vi "数据表比对.vi"(6 "table输入 3":string(combo), 8 "error in (no error)":errorcluster, 9 "table输入 2":string(combo), 10 "仪器日志参数":string, 11 "table输入":string(combo)) -> (0 "error out":errorcluster, 2 "待发送第一条数据":string[](array[string]), 3 "待发送数据":string[][](table), 4 "获取有效数据":string[][](array[string]))   [LabVIEW 2016]
panel:
  out "获取有效数据 3":string[][](array[string])
  out "获取有效数据 2":string[][](array[string])
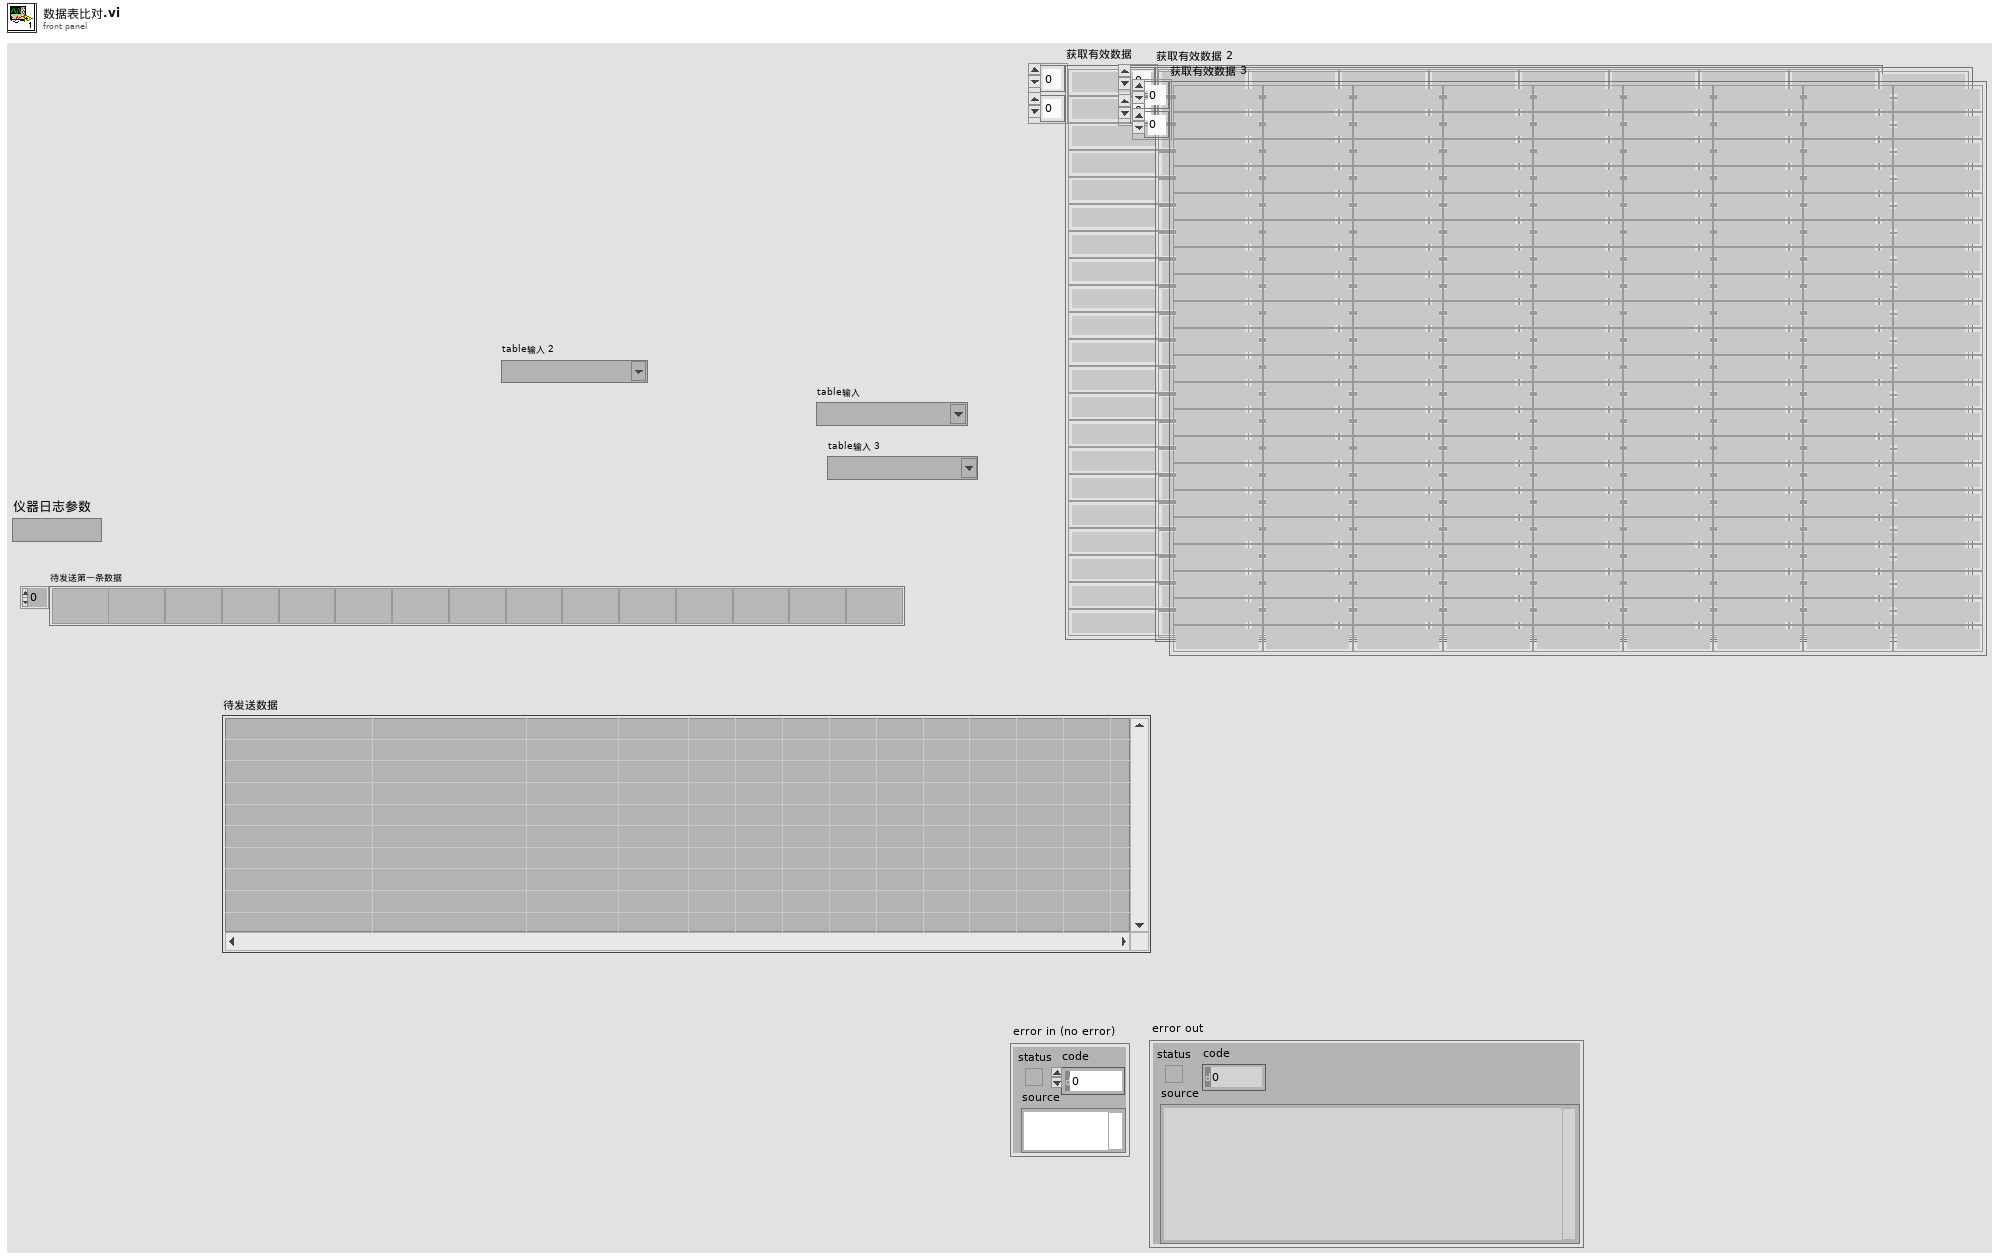
[diagram p1: front panel]
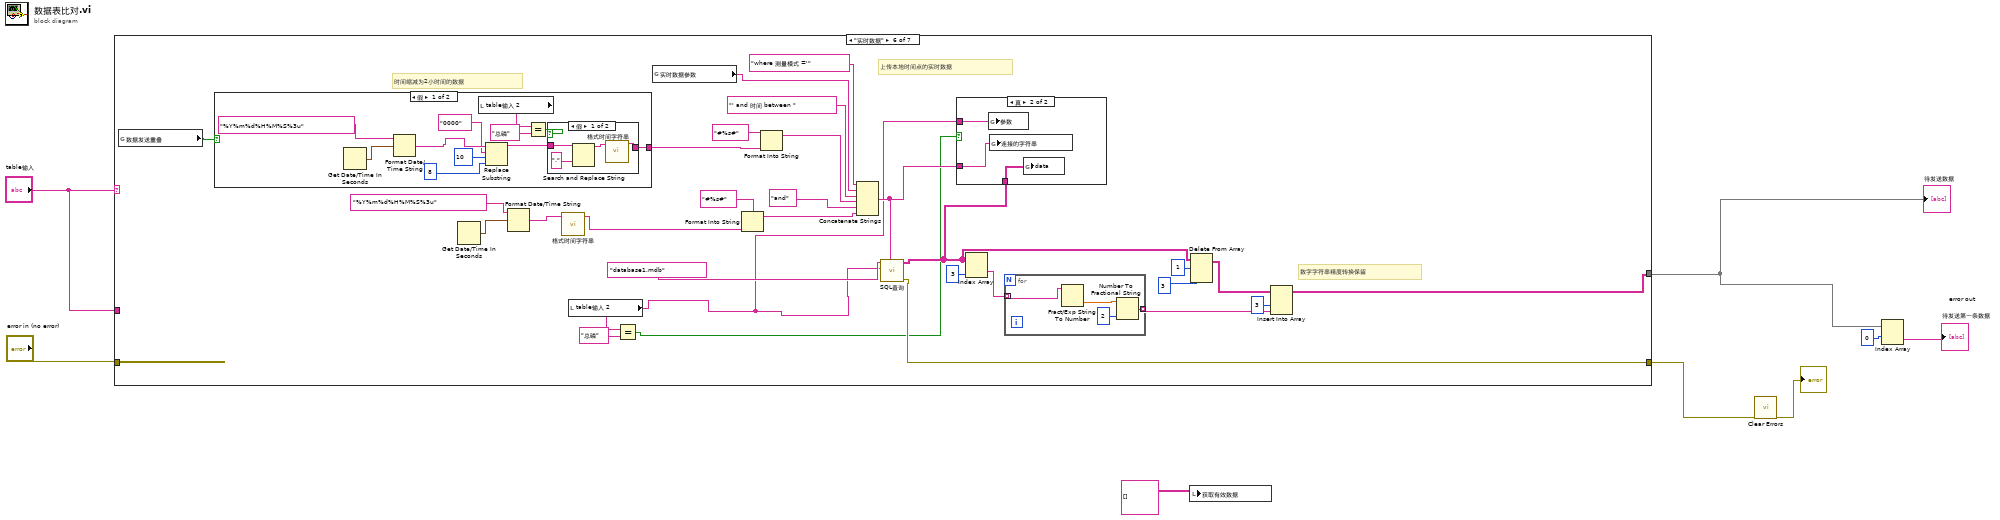
[diagram p0: block diagram]
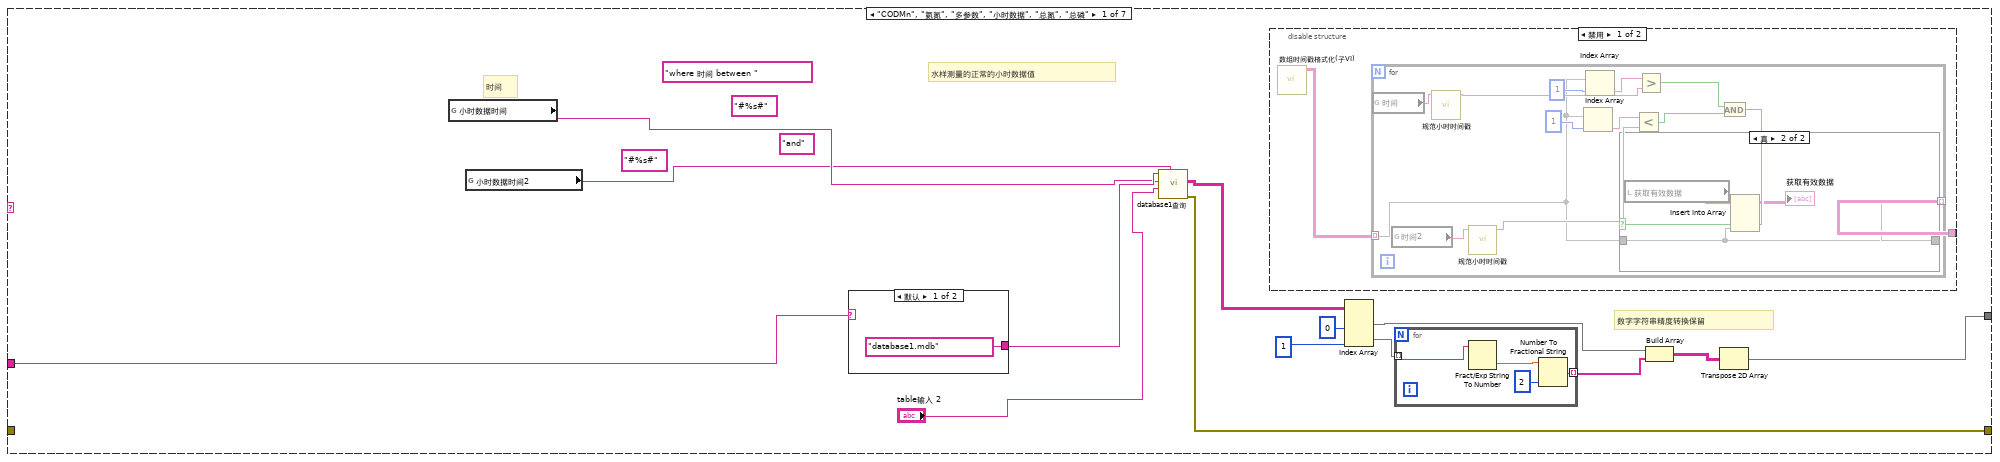
[diagram p2: hidden frame]
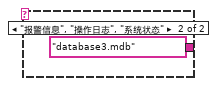
[diagram p5: hidden frame]
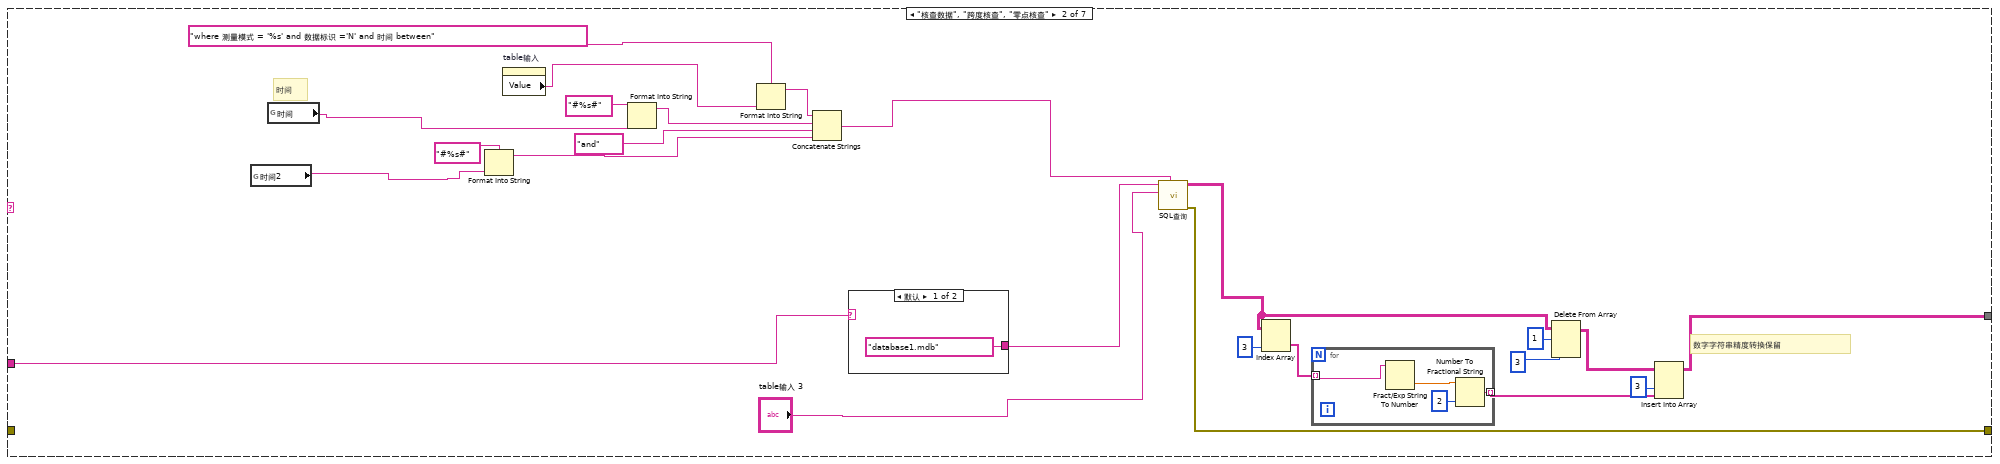
[diagram p6: hidden frame]
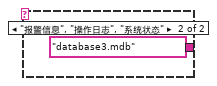
[diagram p7: hidden frame]
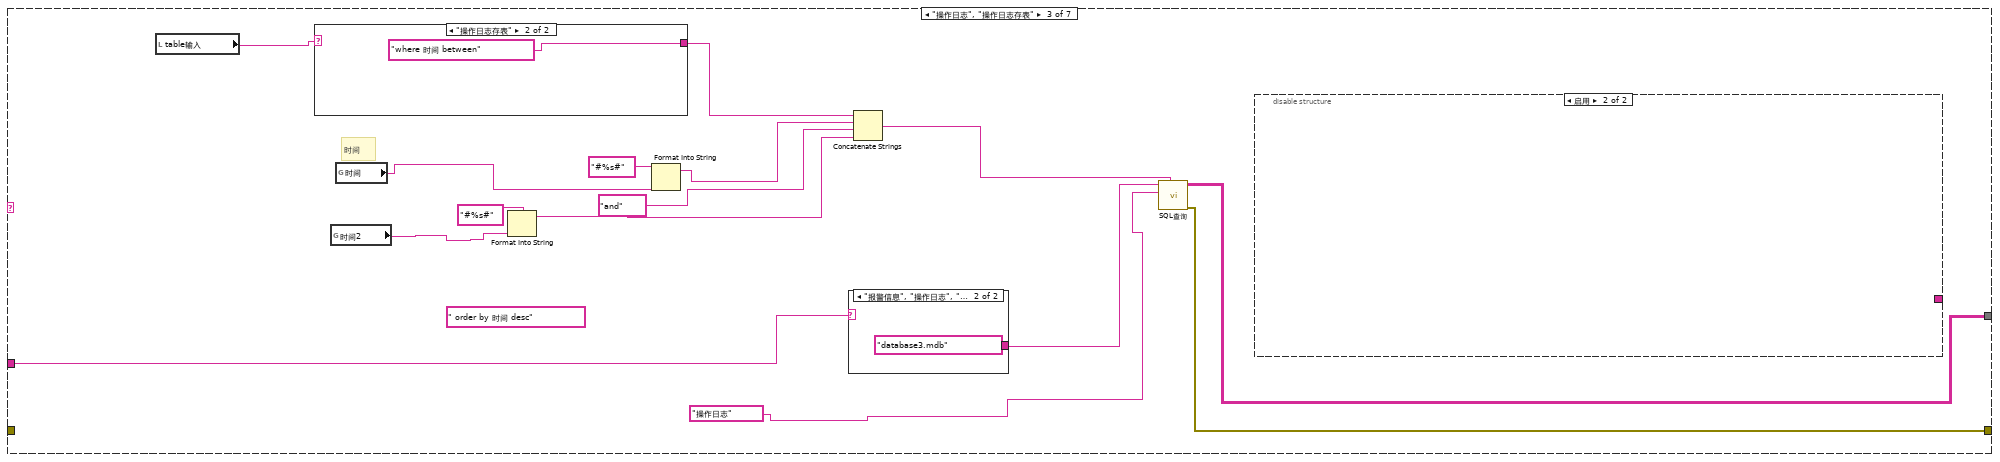
[diagram p8: hidden frame]
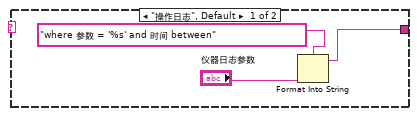
[diagram p9: hidden frame]
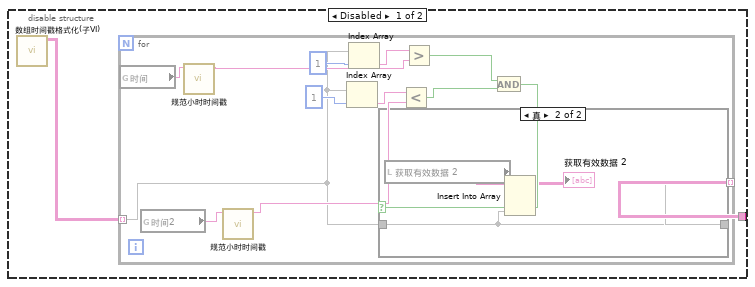
[diagram p10: hidden frame]
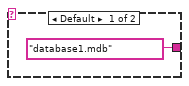
[diagram p12: hidden frame]
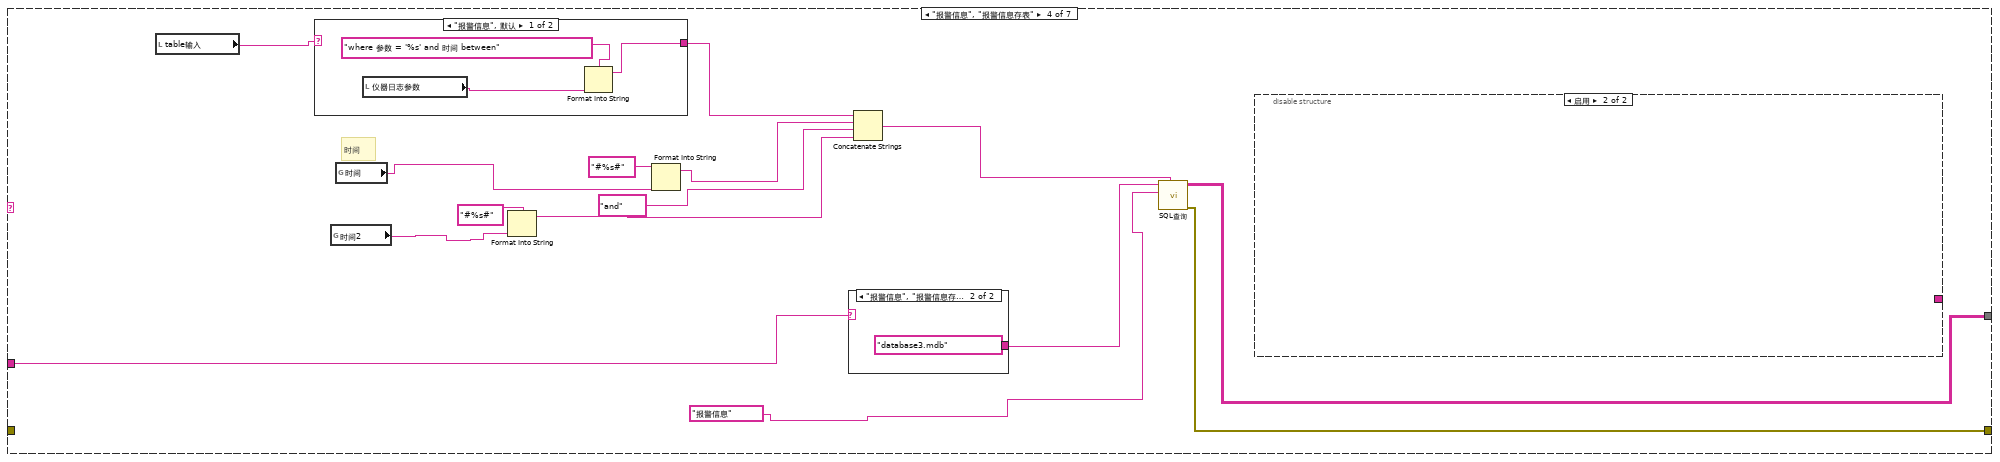
[diagram p13: hidden frame]
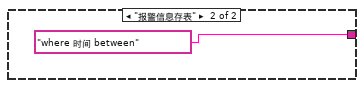
[diagram p14: hidden frame]
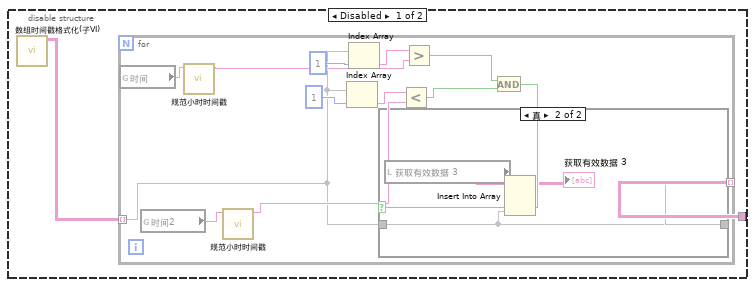
[diagram p15: hidden frame]
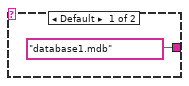
[diagram p17: hidden frame]
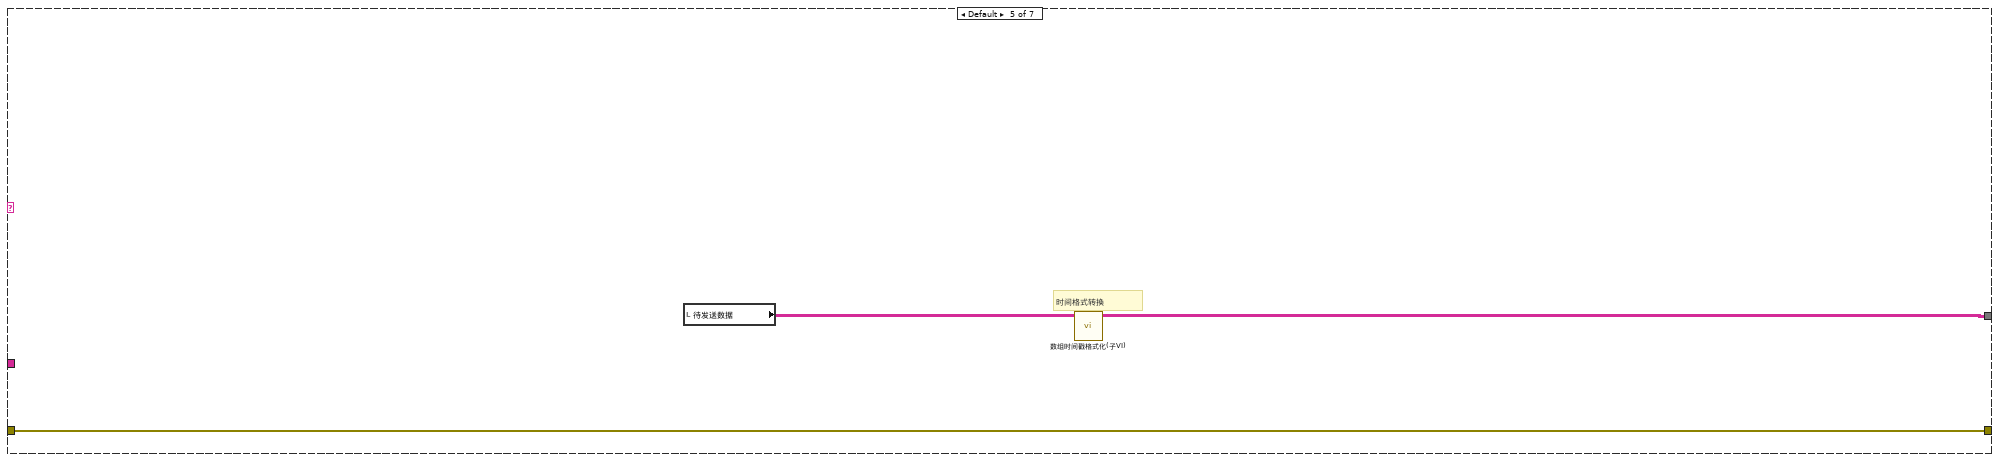
[diagram p18: hidden frame]
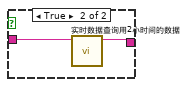
[diagram p20: hidden frame]
diagram:
  n1 = case shown="\"实时数据\"" "table输入" {
    tunnel: "error in (no error)" -> [_ _ _ _ w157 _ _]
    tunnel: [w19 w68 w89 w128 w157 w183 w221] -> w6
    tunnel: [w9 w47 w87 w126 w155 w165 w212] -> w2
    tunnel: "table输入" -> [w22 w70 w91 w130 _ _ _]
    frame "CODMn", "氨氮", "多参数", "小时数据", "总氮", "总磷" {
      (unwired) "and" ("字符串")
      (unwired) "#%s#" ("初始字符串")
      (unwired) "#%s#" ("初始字符串")
      (unwired) "where 时间 between " ("condition")
      # "数字字符串精度转换保留"
      # "水样测量的正常的小时数据值"
      # "时间"
      n2 = global read "全局 时间.vi" "小时数据时间"() -> (w18:string)
      n3 = global read "全局 时间2.vi" "小时数据时间2"() -> (w17:string)
      n4 = case shown="默认" w22 {
        tunnel: ["database1.mdb" ("database") "database3.mdb" ("database")] -> w21
        frame Default {
        }
        frame "报警信息", "操作日志", "系统状态" {
        }
      }
      n5 = call "database1查询.vi"("时间2"=w17, "table"="table输入 2", "时间1"=w18, "database"=w21) -> ("error out"=w19:errorcluster, "data"=w16:string[][])  [unwired: 4 in, 1 out]
      n6 = disable-structure shown="禁用" {
        disable-tunnel: [w27 _] -> _
        frame Disabled {
          n7 = call "数组时间戳格式化(子VI).vi"() -> ("待发送数据输出"=w28:string[][])  [unwired: 11 in]
          n8 = for {
            tunnel: w28 -> [w29] mode=indexing
            tunnel: [w31] -> w27 mode=indexing
            n9 = global read "全局 时间.vi" "时间"() -> (w35:string)
            n10 = global read "全局 时间2.vi" "时间2"() -> (w33:string)
            n11 = call "规范小时时间戳.vi"("字符串"=w35) -> ("result string"=w34:string)  [unwired: 10 in]
            n12 = call "规范小时时间戳.vi"("字符串"=w33) -> ("result string"=w32:string)  [unwired: 10 in]
            n13 = Index Array(array=w29, index=1 ("索引")) -> (element=w38:string)
            n14 = Index Array(array=w29, index=1 ("索引")) -> (element=w40:string)
            n15 = Less?(x=w38, y=w32) -> (x < y?=w37:bool)
            n16 = Greater?(x=w40, y=w34) -> (0:w36:bool)
            n17 = And(x=w36, y=w37) -> (x .and. y?=w30:bool)
            n18 = case shown="真" w30 {
              tunnel: w29 -> [_ w44]
              tunnel: [_ w44] -> w31
              frame False {
              }
              frame True {
                n19 = local read "获取有效数据"() -> (w43:string[][])
                n20 = Insert Into Array(array=w43, new element=w44) -> (→"获取有效数据":string[][])  [unwired: 2 in]
              }
            }
          }
        }
        frame Enabled {
        }
      }
      n21 = Index Array(array=w16, index (col) #1=0 ("禁用的索引 (列)"), index (col) #2=1 ("索引 (列)")) -> (element #1=w12:string[], element #2=w13:string[])  [unwired: 2 in]
      n22 = for {
        tunnel: w13 -> [w24] mode=indexing
        tunnel: [w23] -> w11 mode=indexing
        n23 = Fract/Exp String To Number(string=w24) -> (number=w25:dbl)  [unwired: 3 in, 1 out]
        n24 = Number To Fractional String(number=w25, precision (6)=i16 2 ("精度(6)")) -> (F-format string=w23:string)  [unwired: 2 in]
      }
      n25 = Build Array(w12, w11) -> (w10:string[][])
      n26 = Transpose 2D Array(2D array=w10) -> (transposed array=w9:string[][])
    }
    frame "核查数据", "跨度核查", "零点核查" {
      # "数字字符串精度转换保留"
      # "时间"
      n27 = global read "全局 时间2.vi" "时间2"() -> (w56:string)
      n28 = global read "全局 时间.vi" "时间"() -> (w57:string)
      n29 = Format Into String(format string="#%s#" ("初始字符串"), w56) -> (resulting string=w63:string)  [unwired: 2 in, 1 out]
      n30 = property on="table输入" class="CmbBox"() -> ("Value"=w59:string)  [unwired: 2 in, 2 out]
      n31 = Format Into String(format string="#%s#" ("初始字符串"), w57) -> (resulting string=w67:string)  [unwired: 2 in, 1 out]
      n32 = Format Into String(format string="where 测量模式 = '%s' and 数据标识 ='N' and 时间 between" ("condition"), w59) -> (resulting string=w61:string)  [unwired: 2 in, 1 out]
      n33 = Concatenate Strings(w61, w67, "and" ("字符串"), w63) -> (w60:string)
      n34 = case shown="默认" w70 {
        tunnel: ["database1.mdb" ("database") "database3.mdb" ("database")] -> w69
        frame Default {
        }
        frame "报警信息", "操作日志", "系统状态" {
        }
      }
      n35 = call "SQL查询.vi"("condition"=w60, "table输入"="table输入 3", "database"=w69) -> ("error out"=w68:errorcluster, "data"=w48:string[][])  [unwired: 7 in]
      n36 = Index Array(array=w48, index (col)=3 ("禁用的索引 (列)")) -> (element=w54:string[])  [unwired: 1 in]
      n37 = for {
        tunnel: w54 -> [w72] mode=indexing
        tunnel: [w71] -> w50 mode=indexing
        n38 = Fract/Exp String To Number(string=w72) -> (number=w73:dbl)  [unwired: 3 in, 1 out]
        n39 = Number To Fractional String(number=w73, precision (6)=i16 2 ("精度(6)")) -> (F-format string=w71:string)  [unwired: 2 in]
      }
      n40 = Delete From Array(array=w48, length=1 ("长度"), index (col)=3 ("禁用的索引 (列)")) -> (array with subset deleted=w51:string[][])  [unwired: 1 in, 1 out]
      n41 = Insert Into Array(array=w51, index (col)=3 ("禁用的索引 (列)"), new element=w50) -> (w47:string[][])  [unwired: 1 in]
    }
    frame "操作日志", "操作日志存表" {
      (unwired) " order by 时间 desc" ("字符串")
      # "时间"
      n42 = local read "table输入"() -> (w79:string)
      n43 = case shown="\"操作日志存表\"" w79 {
        tunnel: [w92 "where 时间 between" ("condition")] -> w78
        frame "操作日志", Default {
          n44 = Format Into String(format string="where 参数 = '%s' and 时间 between" ("condition"), "仪器日志参数") -> (resulting string=w92:string)  [unwired: 2 in, 1 out]
        }
        frame "操作日志存表" {
        }
      }
      n45 = global read "全局 时间2.vi" "时间2"() -> (w80:string)
      n46 = global read "全局 时间.vi" "时间"() -> (w81:string)
      n47 = Format Into String(format string="#%s#" ("初始字符串"), w80) -> (resulting string=w82:string)  [unwired: 2 in, 1 out]
      n48 = Format Into String(format string="#%s#" ("初始字符串"), w81) -> (resulting string=w86:string)  [unwired: 2 in, 1 out]
      n49 = case shown="\"报警信息\", \"操作日志\", \"操作日志存表\", \"系统状态\"" w91 {
        tunnel: ["database1.mdb" ("database") "database3.mdb" ("database")] -> w90
        frame Default {
        }
        frame "报警信息", "操作日志", "操作日志存表", "系统状态" {
        }
      }
      n50 = Concatenate Strings(w78, w86, "and" ("字符串"), w82) -> (w88:string)
      n51 = call "SQL查询.vi"("condition"=w88, "table输入"="操作日志", "database"=w90) -> ("error out"=w89:errorcluster, "data"=w87:string[][])  [unwired: 7 in]
      n52 = disable-structure shown="启用" {
        disable-tunnel: [w96 _] -> _
        frame Disabled {
          n53 = call "数组时间戳格式化(子VI).vi"() -> ("待发送数据输出"=w97:string[][])  [unwired: 11 in]
          n54 = for {
            tunnel: w97 -> [w98] mode=indexing
            tunnel: [w100] -> w96 mode=indexing
            n55 = global read "全局 时间.vi" "时间"() -> (w104:string)
            n56 = global read "全局 时间2.vi" "时间2"() -> (w102:string)
            n57 = call "规范小时时间戳.vi"("字符串"=w104) -> ("result string"=w103:string)  [unwired: 10 in]
            n58 = call "规范小时时间戳.vi"("字符串"=w102) -> ("result string"=w101:string)  [unwired: 10 in]
            n59 = Index Array(array=w98, index=1 ("索引")) -> (element=w107:string)
            n60 = Index Array(array=w98, index=1 ("索引")) -> (element=w109:string)
            n61 = Less?(x=w107, y=w101) -> (x < y?=w106:bool)
            n62 = Greater?(x=w109, y=w103) -> (0:w105:bool)
            n63 = And(x=w105, y=w106) -> (x .and. y?=w99:bool)
            n64 = case shown="真" w99 {
              tunnel: w98 -> [_ w113]
              tunnel: [_ w113] -> w100
              frame False {
              }
              frame True {
                n65 = local read "获取有效数据 2"() -> (w112:string[][])
                n66 = Insert Into Array(array=w112, new element=w113) -> (→"获取有效数据 2":string[][])  [unwired: 2 in]
              }
            }
          }
        }
        frame Enabled {
        }
      }
    }
    frame "报警信息", "报警信息存表" {
      # "时间"
      n67 = local read "table输入"() -> (w118:string)
      n68 = case shown="\"报警信息\", 默认" w118 {
        tunnel: [w132 "where 时间 between" ("condition")] -> w117
        frame "报警信息", Default {
          n69 = local read "仪器日志参数"() -> (w131:string)
          n70 = Format Into String(format string="where 参数 = '%s' and 时间 between" ("condition"), w131) -> (resulting string=w132:string)  [unwired: 2 in, 1 out]
        }
        frame "报警信息存表" {
        }
      }
      n71 = global read "全局 时间2.vi" "时间2"() -> (w119:string)
      n72 = global read "全局 时间.vi" "时间"() -> (w120:string)
      n73 = Format Into String(format string="#%s#" ("初始字符串"), w119) -> (resulting string=w121:string)  [unwired: 2 in, 1 out]
      n74 = Format Into String(format string="#%s#" ("初始字符串"), w120) -> (resulting string=w125:string)  [unwired: 2 in, 1 out]
      n75 = case shown="\"报警信息\", \"报警信息存表\", \"操作日志\", \"系统状态\"" w130 {
        tunnel: ["database1.mdb" ("database") "database3.mdb" ("database")] -> w129
        frame Default {
        }
        frame "报警信息", "报警信息存表", "操作日志", "系统状态" {
        }
      }
      n76 = Concatenate Strings(w117, w125, "and" ("字符串"), w121) -> (w127:string)
      n77 = call "SQL查询.vi"("condition"=w127, "table输入"="报警信息", "database"=w129) -> ("error out"=w128:errorcluster, "data"=w126:string[][])  [unwired: 7 in]
      n78 = disable-structure shown="启用" {
        disable-tunnel: [w135 _] -> _
        frame Disabled {
          n79 = call "数组时间戳格式化(子VI).vi"() -> ("待发送数据输出"=w136:string[][])  [unwired: 11 in]
          n80 = for {
            tunnel: w136 -> [w137] mode=indexing
            tunnel: [w139] -> w135 mode=indexing
            n81 = global read "全局 时间.vi" "时间"() -> (w143:string)
            n82 = global read "全局 时间2.vi" "时间2"() -> (w141:string)
            n83 = call "规范小时时间戳.vi"("字符串"=w143) -> ("result string"=w142:string)  [unwired: 10 in]
            n84 = call "规范小时时间戳.vi"("字符串"=w141) -> ("result string"=w140:string)  [unwired: 10 in]
            n85 = Index Array(array=w137, index=1 ("索引")) -> (element=w146:string)
            n86 = Index Array(array=w137, index=1 ("索引")) -> (element=w148:string)
            n87 = Less?(x=w146, y=w140) -> (x < y?=w145:bool)
            n88 = Greater?(x=w148, y=w142) -> (0:w144:bool)
            n89 = And(x=w144, y=w145) -> (x .and. y?=w138:bool)
            n90 = case shown="真" w138 {
              tunnel: w137 -> [_ w152]
              tunnel: [_ w152] -> w139
              frame False {
              }
              frame True {
                n91 = local read "获取有效数据 3"() -> (w151:string[][])
                n92 = Insert Into Array(array=w151, new element=w152) -> (→"获取有效数据 3":string[][])  [unwired: 2 in]
              }
            }
          }
        }
        frame Enabled {
        }
      }
    }
    frame Default {
      # "时间格式转换"
      n93 = local read "待发送数据"() -> (w156:string[][])
      n94 = call "数组时间戳格式化(子VI).vi"("待发送数据输入"=w156) -> ("待发送数据输出"=w155:string[][])  [unwired: 10 in]
    }
    frame "实时数据" {
      # "时间缩减为2小时间的数据"
      # "数字字符串精度转换保留"
      # "上传本地时间点的实时数据"
      n95 = global read "全局 数据发送重叠.vi" "数据发送重叠"() -> (w164:bool)
      n96 = case shown="假" w164 {
        tunnel: [w193 w207] -> w182
        frame False {
          n97 = Get Date/Time In Seconds() -> (seconds since 1Jan1904=w200:timestamp)
          n98 = Format Date/Time String(time format string (%c)="%Y%m%d%H%M%S%3u" ("时间格式字符串(%c)"), seconds (now)=w200) -> (date/time string=w198:string)  [unwired: 1 in]
          n99 = local read "table输入 2"() -> (w192:string)
          n100 = Replace Substring(2:8 ("长度（子字符串长度）"), 3:10 ("偏移量(0)"), 4:"0000" ("子字符串(\"\")"), 5:w198) -> (1:w194:string)  [unwired: 1 out]
          n101 = Equal?(x=w192, y="总磷") -> (x = y?=w190:bool)
          n102 = case shown="假" w190 {
            tunnel: w194 -> [w202 w206]
            tunnel: [w201 w205] -> w193
            frame False {
              n103 = Search and Replace String(input string=w202, search string="." ("搜索字符串")) -> (result string=w203:string)  [unwired: 6 in, 3 out]
              n104 = call "格式时间字符串.vi"("字符串"=w203) -> ("连接的字符串"=w201:string)  [unwired: 10 in]
            }
            frame True {
              n105 = call "实时数据查询用2小时间的数据.vi"("字符串"=w206) -> ("连接的字符串"=w205:string)  [unwired: 10 in]
            }
          }
        }
        frame True {
          n106 = global read "全局 数据发送重叠.vi" "数据发送重叠开始时间戳"() -> (w207:string)
        }
      }
      n107 = Get Date/Time In Seconds() -> (seconds since 1Jan1904=w178:timestamp)
      n108 = Format Date/Time String(time format string (%c)="%Y%m%d%H%M%S%3u" ("时间格式字符串(%c)"), seconds (now)=w178) -> (date/time string=w176:string)  [unwired: 1 in]
      n109 = call "格式时间字符串.vi"("字符串"=w176) -> ("连接的字符串"=w175:string)  [unwired: 10 in]
      n110 = local read "table输入 2"() -> (w160:string)
      n111 = Equal?(x=w160, y="总磷") -> (x = y?=w159:bool)
      n112 = global read "全局 实时数据参数.vi" "实时数据参数"() -> (w158:string)
      n113 = Format Into String(format string="#%s#" ("初始字符串"), w175) -> (resulting string=w180:string)  [unwired: 2 in, 1 out]
      n114 = Format Into String(format string="#%s#" ("初始字符串"), w182) -> (resulting string=w186:string)  [unwired: 2 in, 1 out]
      n115 = Concatenate Strings("where 测量模式 ='" ("condition"), w158, "' and 时间 between ", w186, "and" ("字符串"), w180) -> (w162:string)
      n116 = call "SQL查询.vi"("condition"=w162, "table输入"=w160, "database"="database1.mdb") -> ("error out"=w183:errorcluster, "data"=w161:string[][])  [unwired: 7 in]
      n117 = case shown="真" w159 {
        tunnel: w162 -> [_ w189]
        tunnel: w161 -> [_ w188]
        tunnel: w160 -> [_ w187]
        frame False {
        }
        frame True {
          n118 = global write "全局 实时数据参数.vi" "参数"(w187) -> ()
          n119 = global write "全局 实时数据参数.vi" "连接的字符串"(w189) -> ()
          n120 = global write "全局 实时数据参数.vi" "data"(w188) -> ()
        }
      }
      n121 = Index Array(array=w161, index (col)=3 ("禁用的索引 (列)")) -> (element=w171:string[])  [unwired: 1 in]
      n122 = for {
        tunnel: w171 -> [w209] mode=indexing
        tunnel: [w208] -> w167 mode=indexing
        n123 = Fract/Exp String To Number(string=w209) -> (number=w210:dbl)  [unwired: 3 in, 1 out]
        n124 = Number To Fractional String(number=w210, precision (6)=i16 2 ("精度(6)")) -> (F-format string=w208:string)  [unwired: 2 in]
      }
      n125 = Delete From Array(array=w161, length=1 ("长度"), index (col)=3 ("禁用的索引 (列)")) -> (array with subset deleted=w168:string[][])  [unwired: 1 in, 1 out]
      n126 = Insert Into Array(array=w168, index (col)=3 ("禁用的索引 (列)"), new element=w167) -> (w165:string[][])  [unwired: 1 in]
    }
    frame "提取实时数据" {
      # "数字字符串精度转换保留"
      # "上传给定时间段之间的实时数据"
      n127 = global read "起始时间.vi" "起始时间"() -> (w223:string)
      n128 = global read "起始时间.vi" "结束时间"() -> (w222:string)
      n129 = local read "table输入 2"() -> (w227:string)
      n130 = Format Into String(format string="#%s#" ("初始字符串"), w223) -> (resulting string=w231:string)  [unwired: 2 in, 1 out]
      n131 = Format Into String(format string="#%s#" ("初始字符串"), w222) -> (resulting string=w224:string)  [unwired: 2 in, 1 out]
      n132 = Concatenate Strings("where 测量模式 ='水样测试' and 时间 between " ("condition"), w231, "and" ("字符串"), w224) -> (w229:string)
      n133 = call "SQL查询.vi"("condition"=w229, "table输入"=w227, "database"="database1.mdb") -> ("error out"=w221:errorcluster, "data"=w218:string[][])  [unwired: 7 in]
      n134 = Index Array(array=w218, index (col)=3 ("禁用的索引 (列)")) -> (element=w219:string[])  [unwired: 1 in]
      n135 = for {
        tunnel: w219 -> [w234] mode=indexing
        tunnel: [w233] -> w214 mode=indexing
        n136 = Fract/Exp String To Number(string=w234) -> (number=w235:dbl)  [unwired: 3 in, 1 out]
        n137 = Number To Fractional String(number=w235, precision (6)=i16 2 ("精度(6)")) -> (F-format string=w233:string)  [unwired: 2 in]
      }
      n138 = Delete From Array(array=w218, length=1 ("长度"), index (col)=3 ("禁用的索引 (列)")) -> (array with subset deleted=w215:string[][])  [unwired: 1 in, 1 out]
      n139 = Insert Into Array(array=w215, index (col)=3 ("禁用的索引 (列)"), new element=w214) -> (w212:string[][])  [unwired: 1 in]
    }
  }
  "待发送数据" <- w2
  n140 = local write "获取有效数据"(string[][] []) -> ()
  n141 = call <vilib>:"Clear Errors.vi"("error in (no error)"=w6) -> ("error out"=→"error out":errorcluster)  [unwired: 5 in, 1 out]
  n142 = Index Array(array=w2, index (row)=0 ("索引 (行)")) -> (element=→"待发送第一条数据":string[])  [unwired: 1 in]
